vi "S2C_FORNAX_Proc_WaitForResponse.vi"(8 "Error In":errorcluster, 11 "Timeout":dbl) -> (0 "Error Out":errorcluster, 3 "Response":string)   [LabVIEW 2015]
uses:
  S2C_FORNAX_Proc_Globals.vi
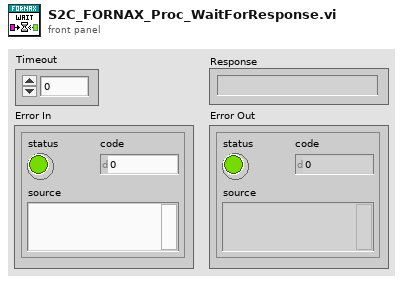
[diagram p1: front panel]
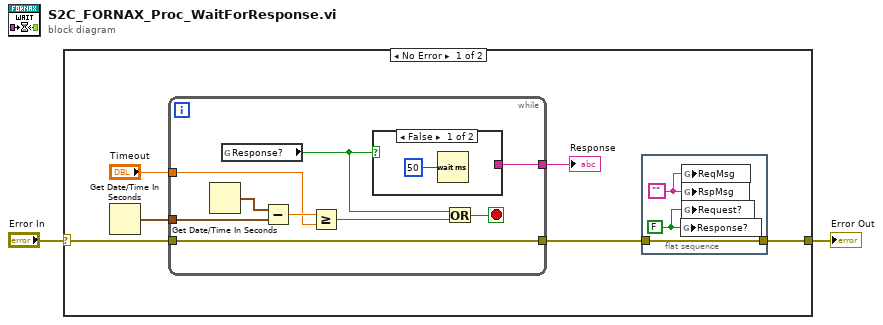
[diagram p0: block diagram]
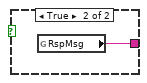
[diagram p2: hidden frame]
diagram:
  n1 = case shown="No Error" "Error In" {
    selector: "Error In" -> [w8 w23]
    tunnel: [w5 w23] -> w1
    frame No Error {
      n2 = Get Date/Time In Seconds() -> (seconds since 1Jan1904=w4:timestamp)
      n3 = while {
        tunnel: w8 -> [w12]
        tunnel: [w12] -> w6
        tunnel: [w20] -> w7
        tunnel: w4 -> [w18]
        tunnel: "Timeout" -> [w16]
        stop <- w13 stop-if-true
        n4 = Get Date/Time In Seconds() -> (seconds since 1Jan1904=w19:timestamp)
        n5 = global read "S2C_FORNAX_Proc_Globals.vi" "Response?"() -> (w15:bool)
        n6 = Subtract(x=w19, y=w18) -> (x-y=w17:dbl)
        n7 = Greater Or Equal?(x=w17, y=w16) -> (x >= y?=w14:bool)
        n8 = case shown="False" w15 {
          tunnel: [_ w22] -> w20
          frame False {
            n9 = Wait (ms)(milliseconds to wait=u32 50) -> ()  [unwired: 1 out]
          }
          frame True {
            n10 = global read "S2C_FORNAX_Proc_Globals.vi" "RspMsg"() -> (w22:string)
          }
        }
        n11 = Or(x=w15, y=w14) -> (x .or. y?=w13:bool)
      }
      "Response" <- w7
      n12 = flat-sequence {
        tunnel: w6 -> [w11]
        tunnel: [w11] -> w5
        frame #0 {
          w9 = FALSE ("Response?")
          w10 = ""
          n13 = global write "S2C_FORNAX_Proc_Globals.vi" "Response?"(w9) -> ()
          n14 = global write "S2C_FORNAX_Proc_Globals.vi" "ReqMsg"(w10) -> ()
          n15 = global write "S2C_FORNAX_Proc_Globals.vi" "RspMsg"(w10) -> ()
          n16 = global write "S2C_FORNAX_Proc_Globals.vi" "Request?"(w9) -> ()
        }
      }
    }
    frame Error {
    }
  }
  "Error Out" <- w1
